vi "fo_LocatePatientInfo.vi"(11 "subarray":string[](array[string])) -> (2 "PatientId":string, 3 "PatientName":string)   [LabVIEW 2013, in "main.lvlib"]
uses:
  main.lvlib
  Controls/Enum Variables.ctl
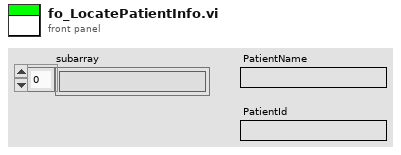
[diagram p1: front panel]
types:
  T1 = typedef "main.lvlib/Enum Variables.ctl" = enum16{"SetAcqFilter", "GetAcqFilter", "Set Filter", "Get Filter", "Set Height", "Get Height", "Set Recorded Height", "Get Recorded Height", "Set Blue Pressure", "Get Blue Pressure", "Set Red Pressure", "Get Red Pressure", "Init", "Reset Pressure", "Set Red Cursors", "Get Red Cursors", "Set Blue Cursors", "Get Blue Cursors", "Set Language", "Get Language", "Set Active Graphs", "Get ActiveGraphs", "Set Method", "Get Method", "Set Encryption", "Get Encryption", "Set ExcelVersion", "Get ExcelVersion", "Set DICOM Avail", "Get DICOM Avail", "Set DICOM Encode", "Get DICOM Encode", "Set JournalExport", "Get JournalExport", "Set Sequence", "Get Sequence", "Set DAQ Connected", "Get DAQ Connected", "Set Current Graph", "Get Current Graph", "Set General Settings", "Get Hyphenation", "Set Arm Calc Method", "Get Arm Calc Method", "Set Dicom Tags", "Get Dicom Tags", "Set BT Serial", "Get BT Serial", "Set BT Accepted Serials", "Get BT Accepted Serials", "Get BT License", "Set BT License"}
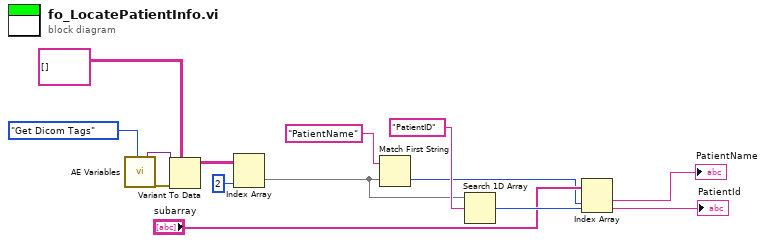
[diagram p0: block diagram]
diagram:
  n1 = call "AE Variables.vi"("Action"=Enum_Variables."Get Dicom Tags") -> ("Variant"=w5:variant, "error out"=w8:errorcluster)  [unwired: 11 in, 6 out]
  n2 = Variant To Data(error in=w8, type=string[][] [], Variant=w5) -> (data=w6:string[][])  [unwired: 1 out]
  n3 = Index Array(array=w6, index (col)=2 ("disabled index (col)")) -> (element=w2:string[])  [unwired: 1 in]
  n4 = Match First String(2:w2, 3:"PatientName" ("element")) -> (0:w1:i32)  [unwired: 1 out]
  n5 = Search 1D Array(1D array=w2, element="PatientID") -> (index of element=w14:i32)  [unwired: 1 in]
  n6 = Index Array(array="subarray", index #1=w1, index #2=w14) -> (element #1=→"PatientName":string, element #2=→"PatientId":string)
